vi "Read.vi"() -> ()   [LabVIEW 2012]
uses:
  Madlib.dll
panel:
  in  "Axis":u32=1
  in  "# data points to average":i32=1 min=1
  in  "Position":dbl format="%.4f"
  in  "Move":bool
  in  "stop":bool
  out "Position Read um":dbl(graph)=0.20766479492187498
  # "This example reads the position of the nanopositioner in\na continous loop."
  # "X = 1\nY = 2\nZ = 3"
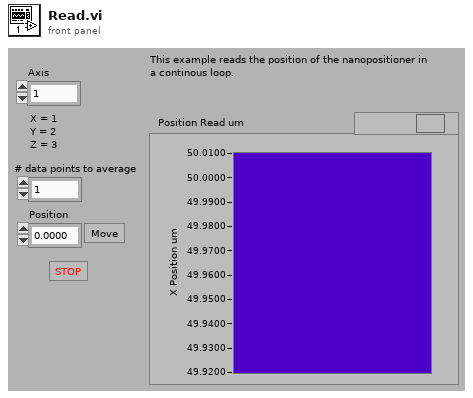
[diagram p1: front panel]
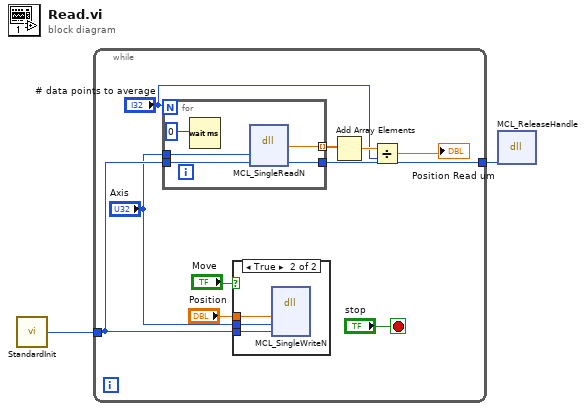
[diagram p0: block diagram]
diagram:
  n1 = call "StandardInit.vi"() -> ("Outgoing Handle"=w1:i32)  [unwired: 1 in]
  n2 = while {
    tunnel: w1 -> [w9]
    tunnel: [w5] -> w2
    stop <- "stop" stop-if-true
    n3 = for {
      N: "# data points to average" -> [_]
      tunnel: w9 -> [w17]
      tunnel: [w15] -> w7 mode=indexing
      tunnel: [w14] -> w5
      tunnel: "Axis" -> [w13]
      n4 = Wait (ms)(milliseconds to wait=0) -> ()  [unwired: 1 out]
      n5 = dll-call lib="C:/Users/Labview/Desktop/SRR/Madlib_x64/Labview Examples/MADLib.dll" fn="MCL_SingleReadN"("axis"=w13, "handle"=w17) -> (w15:dbl, "handle"=w14:i32)  [unwired: 4 in, 2 out]
    }
    n6 = case shown="True" "Move" {
      tunnel: "Position" -> [_ w20]
      tunnel: w9 -> [_ w19]
      tunnel: "Axis" -> [_ w18]
      frame False {
      }
      frame True {
        n7 = dll-call lib="C:/Users/Labview/Desktop/SRR/Madlib_x64/Labview Examples/MADLib.dll" fn="MCL_SingleWriteN"("position"=w20, "axis"=w18, "handle"=w19) -> ()  [unwired: 7 in, 2 out]
      }
    }
    n8 = Add Array Elements(numeric array=w7) -> (sum=w8:dbl)
    n9 = Divide(x=w8, y="# data points to average") -> (x/y=→"Position Read um":dbl)
  }
  n10 = dll-call lib="C:/Users/Labview/Desktop/SRR/Madlib_x64/Labview Examples/MADLib.dll" fn="MCL_ReleaseHandle"("handle"=w2) -> ()  [unwired: 5 in, 2 out]
